vi "4Pi Focus Lock - Setup Camera.vi"(0 "Camera Notifier Name":string) -> (8 "Canceled?":bool)   [LabVIEW 2016]
uses:
  <vilib>/Utility/miscctls.llb/LVPointTypeDef.ctl
  Device Library/Cameras/Camera Controls/Generic Camera ROI.ctl
  Device Library/Cameras/Camera Controls/Generic Camera Actions.ctl
  4Pi Focus Lock Controls/4Pi Focus Lock - Camera Settings.ctl
panel:
  out "ROI Size":string
  in  "Exposure Time (ms)":dbl
  in  "Tool Selection":enum32{"Zoom Tool", "ROI Tool", "Pan Tool"}(radio)
  in  "Cancel":bool
  in  "Done":bool
  out "Camera Display":T1(plugin-control)
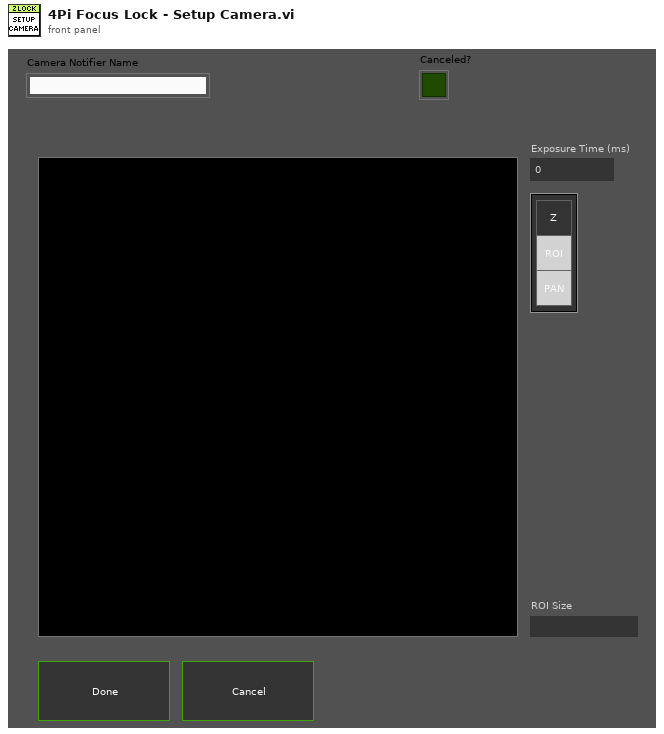
[diagram p1: front panel]
types:
  T1 = typedef "IMAQ Image.ctl" = refnum<image>
  T2 = typedef "Generic Camera Actions.ctl" = enum16{"Status", "Live Preview", "Capture", "Abort", "Set Exposure Time (s)", "Get Exposure Time (s)", "Record Settings", "Set ROI", "Get ROI", "Defect Correction On/Off", "Cooler On/Off", "Fan On/Off", "Quit"}
  T3 = typedef "Generic Camera ROI.ctl" = cluster{"H_Offset":u16, "V_Offset":u16, "H_Width":u16, "V_Width":u16}
  T4 = enum16{"Always On", "Always Off", "Off While Running"}
  T5 = typedef "LVPointTypeDef.ctl" = cluster{"Horizontal":i16, "Vertical":i16}
  T6 = typedef "LVRectTypeDef.ctl" = cluster{"Left":i16, "Top":i16, "Right":i16, "Bottom":i16}
  T7 = typedef "LVBoundsTypeDef.ctl" = cluster{"Width":u32, "Height":u32}
  T8 = typedef "4Pi Focus Lock - Camera Settings.ctl" = cluster{"Exposure Time (s)":dbl, "H Offset":u16, "V Offset":u16, "H Width":u16, "V Width":u16}
  T9 = cluster{"Global Rectangle":i32[], "Contours":cluster{"Contour Type":u32, "ROI Type":u32, "Points":i32[]}[]}
  T10 = cluster{"Contour Type":u32, "ROI Type":u32, "Points":i32[]}[]
  T11 = cluster{"Contour Type":u32, "ROI Type":u32, "Points":i32[]}
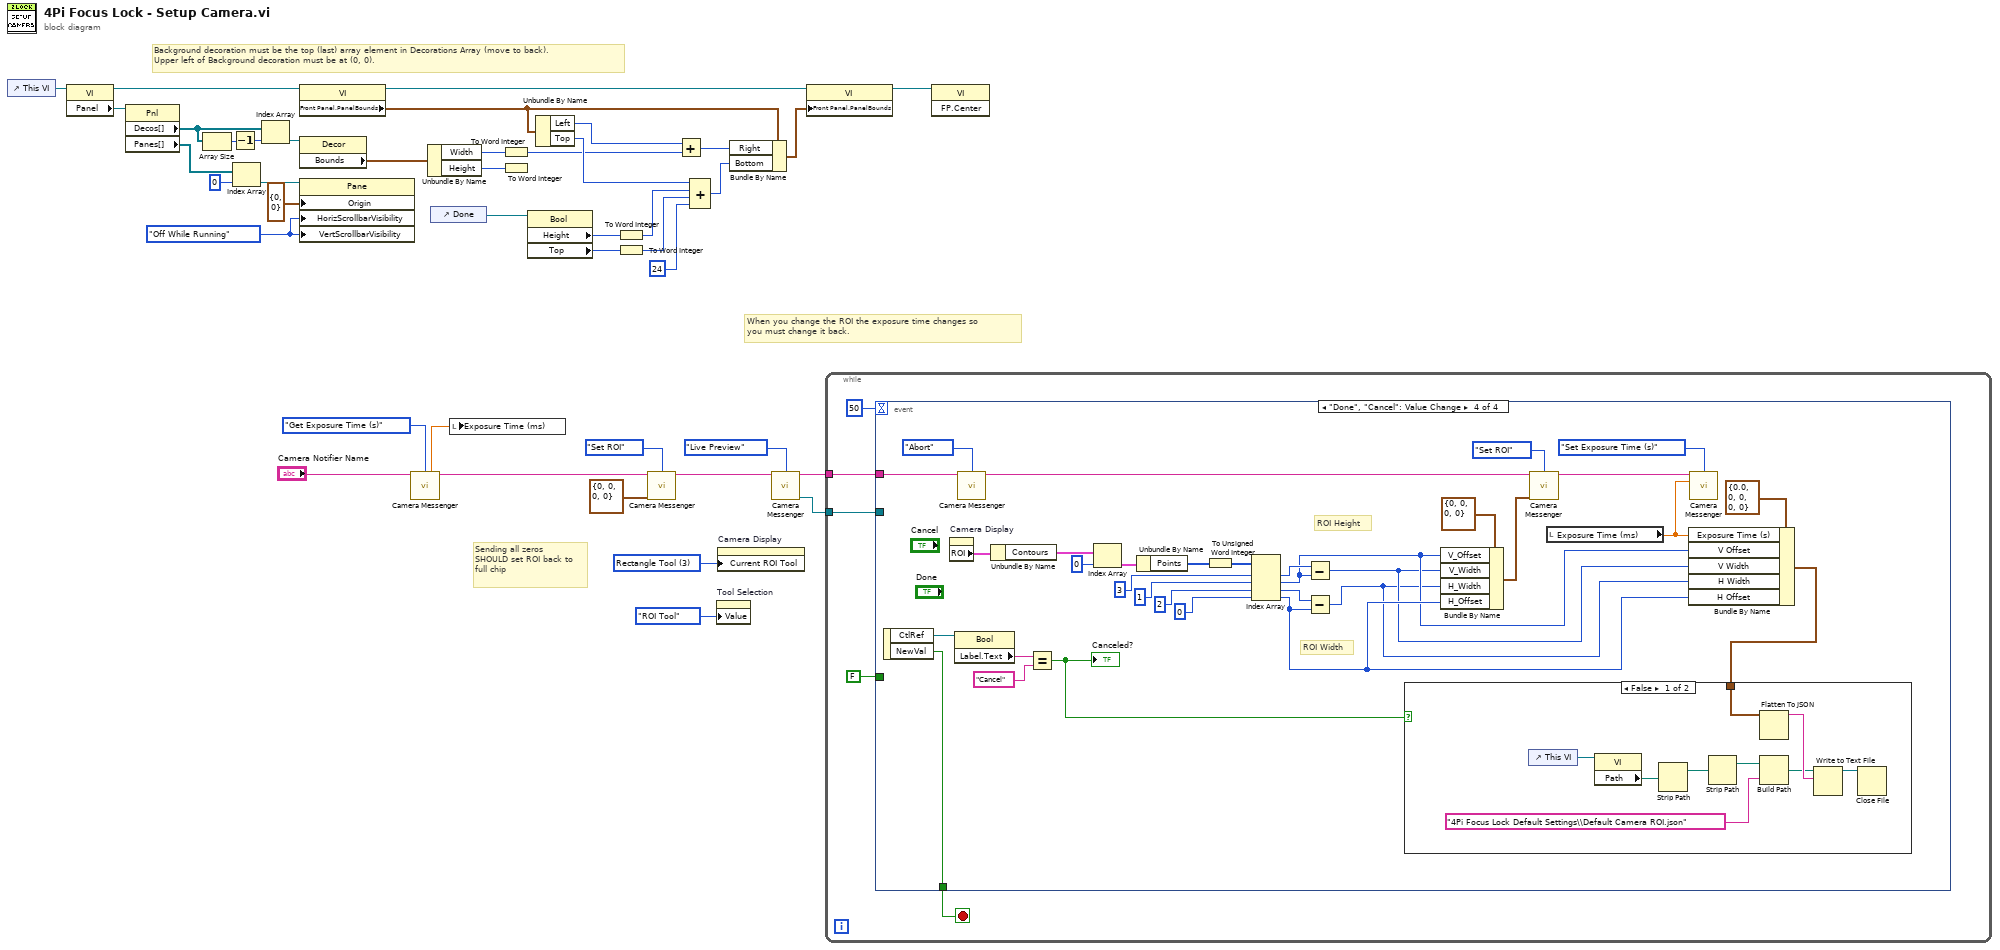
[diagram p0: block diagram]
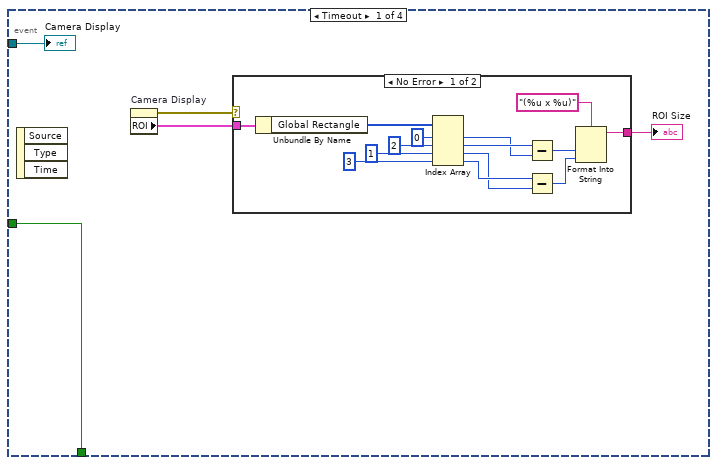
[diagram p2: hidden frame]
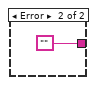
[diagram p3: hidden frame]
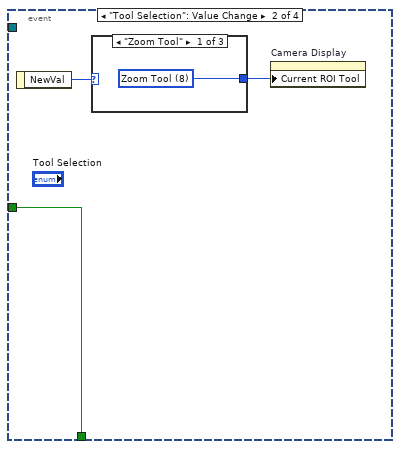
[diagram p4: hidden frame]
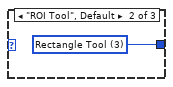
[diagram p5: hidden frame]
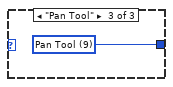
[diagram p6: hidden frame]
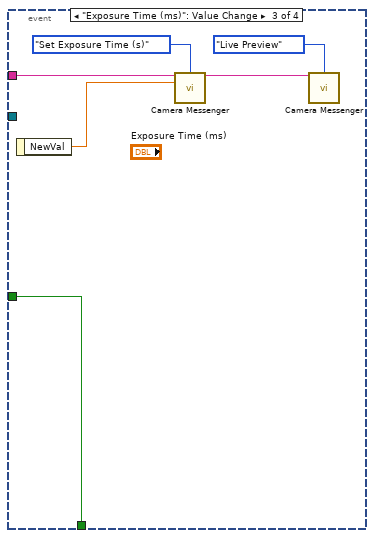
[diagram p7: hidden frame]
diagram:
  w23 = T4."Off While Running" ("Vertical Scrollbar Visibility")
  w42 = u32 3 items=["Zoom Tool"=8, "Selection Tool"=0, "Pan Tool"=9, "Point Tool"=1, "Line Tool"=2, "Rectangle Tool"=3, "Rotated Rectangle Tool"=12, "Polyline Tool"=10, "Polygon Tool"=5, "Freehand Tool"=11, "Closed Freehand Tool"=6, "Ellipse Tool"=4, "Annulus Tool"=7] ("Current ROI Tool")
  # "Background decoration must be the top (last) array element in Decorations Array (move to back).\nUpper left of Background decoration must be at (0, 0)."
  # "When you change the ROI the exposure time changes so\nyou must change it back."
  # "Sending all zeros SHOULD set ROI back to full chip"
  n1 = control-ref of="This VI"() -> (w15:refnum<vi>)
  n2 = property class="VI"(reference=w15) -> (reference out=w24:refnum<vi>, "Panel"=w16:refnum<vi>)  [unwired: 1 in, 1 out]
  n3 = property class="Pnl"(reference=w16) -> ("Decos[]"=w14:refnum<vi>[], "Panes[]"=w20:refnum<vi>[])  [unwired: 1 in, 2 out]
  n4 = Array Size(array=w14) -> (size(s)=w12:i32)
  n5 = Decrement(x=w12) -> (x-1=w13:i32)
  n6 = Index Array(array=w20, index=0) -> (element=w19:refnum<vi>)
  n7 = Index Array(array=w14, index=w13) -> (element=w22:refnum<vi>)
  n8 = property class="VI"(reference=w24) -> (reference out=w26:refnum<vi>, "Front Panel.PanelBounds"=w27:T6)  [unwired: 1 in, 1 out]
  n9 = property class="Decor"(reference=w22) -> ("Bounds"=w25:T7)  [unwired: 1 in, 2 out]
  n10 = property class="Pane"(reference=w19, "Origin"=T5 {"Horizontal"=0, "Vertical"=0}, "HorizScrollbarVisibility"=w23, "VertScrollbarVisibility"=w23) -> ()  [unwired: 1 in, 2 out]
  n11 = call "Camera Messenger.vi"("Notifier Name"="Camera Notifier Name", "General Camera Actions"=Generic_Camera_Actions."Get Exposure Time (s)") -> ("Current Exposure Time (s)"=w8:dbl, "Notifier Name Dup"=w7:string)  [unwired: 8 in, 4 out]
  n12 = Unbundle By Name(w25) -> ("Width"=w30:u32, "Height"=w33:u32)
  n13 = control-ref of="Done"() -> (w17:refnum<vi>)
  n14 = local write "Exposure Time (ms)"(w8) -> ()
  n15 = To Word Integer(number=w30) -> (16bit integer=w32:i16)
  n16 = To Word Integer(number=w33) -> ()  [unwired: 1 out]
  n17 = property class="Bool"(reference=w17) -> ("Height"=w35:u32, "Top"=w36:i32)  [unwired: 1 in, 2 out]
  n18 = Unbundle By Name(w27) -> ("Left"=w29:i16, "Top"=w40:i16)
  n19 = To Word Integer(number=w35) -> (16bit integer=w38:i16)
  n20 = To Word Integer(number=w36) -> (16bit integer=w39:i16)
  n21 = call "Camera Messenger.vi"("Notifier Name"=w7, "General Camera Actions"=Generic_Camera_Actions."Set ROI", "Camera ROI"=T3 {"H_Offset"=0, "V_Offset"=0, "H_Width"=0, "V_Width"=0} ("General Camera ROI")) -> ("Notifier Name Dup"=w4:string)  [unwired: 7 in, 5 out]
  n22 = Add(x=w29, y=w32) -> (x+y=w31:i16)
  n23 = Compound Arithmetic op=ADD(w40, w38, w39, i16 24 ("y")) -> (w34:i16)
  n24 = property on="Tool Selection" class="RadioBtnsControl (strict)"("Value"=enum32{"Zoom Tool", "ROI Tool", "Pan Tool"}."ROI Tool" ("Tool Selection")) -> ()  [unwired: 2 in, 2 out]
  n25 = property on="Camera Display" class="ImageControl"("Current ROI Tool"=w42) -> ()  [unwired: 2 in, 2 out]
  n26 = Bundle By Name(cluster=w27, "Right"=w31, "Bottom"=w34) -> (w28:T6)
  n27 = call "Camera Messenger.vi"("Notifier Name"=w4, "General Camera Actions"=Generic_Camera_Actions."Live Preview") -> ("Notifier Name Dup"=w3:string, "Image Ref"=w1:T1)  [unwired: 8 in, 4 out]
  n28 = property class="VI"(reference=w26, "Front Panel.PanelBounds"=w28) -> (reference out=w11:refnum<vi>)  [unwired: 1 in, 1 out]
  n29 = while {
    tunnel: w1 -> [w45]
    tunnel: w3 -> [w43]
    stop <- w47 stop-if-true
    n30 = event shown="[3] \"Done\", \"Cancel\": Value Change" {
      selector: _ -> [_ _ _ _]
      dyn-events: _ -> [_ _ _ _]
      timeout: 50 -> [_ _ _ _]
      tunnel: [w52 w70 w79 w108] -> w47
      tunnel: FALSE -> [w52 w70 w79 _]
      tunnel: w45 -> [w51 _ _ _]
      tunnel: w43 -> [_ _ w78 w96]
      event Timeout {
        n31 = event-data() -> ()  [unwired: 1 in, 3 out]
        n32 = property on="Camera Display" class="ImageControl"() -> (error out=w49:errorcluster, "ROI"=w50:T9)  [unwired: 2 in, 1 out]
        n33 = case shown="No Error" w49 {
          tunnel: w50 -> [w57 _]
          tunnel: [w53 ""] -> w48
          frame No Error {
            n34 = Unbundle By Name(w57) -> ("Global Rectangle"=w66:i32[])
            n35 = Index Array(array=w66, index #1=0 ("index"), index #2=2 ("index"), index #3=1 ("index"), index #4=3 ("index")) -> (element #1=w60:i32, element #2=w61:i32, element #3=w58:i32, element #4=w59:i32)
            n36 = Subtract(x=w61, y=w60) -> (x-y=w55:i32)
            n37 = Subtract(x=w59, y=w58) -> (x-y=w54:i32)
            n38 = Format Into String(format string="(%u x %u)", w55, w54) -> (resulting string=w53:string)  [unwired: 2 in, 1 out]
          }
          frame Error {
          }
        }
        "ROI Size" <- w48
        "Camera Display" <- w51
      }
      event "Tool Selection": Value Change {
        n39 = event-data() -> ("NewVal"=w69:enum32{"Zoom Tool", "ROI Tool", "Pan Tool"})  [unwired: 1 in]
        n40 = case shown="\"Zoom Tool\"" w69 {
          tunnel: [w71 w72 w73] -> w68
          frame "Zoom Tool" {
            w71 = u32 8 items=["Zoom Tool"=8, "Selection Tool"=0, "Pan Tool"=9, "Point Tool"=1, "Line Tool"=2, "Rectangle Tool"=3, "Rotated Rectangle Tool"=12, "Polyline Tool"=10, "Polygon Tool"=5, "Freehand Tool"=11, "Closed Freehand Tool"=6, "Ellipse Tool"=4, "Annulus Tool"=7] ("Current ROI Tool")
          }
          frame "ROI Tool", Default {
            w72 = u32 3 items=["Zoom Tool"=8, "Selection Tool"=0, "Pan Tool"=9, "Point Tool"=1, "Line Tool"=2, "Rectangle Tool"=3, "Rotated Rectangle Tool"=12, "Polyline Tool"=10, "Polygon Tool"=5, "Freehand Tool"=11, "Closed Freehand Tool"=6, "Ellipse Tool"=4, "Annulus Tool"=7] ("Current ROI Tool")
          }
          frame "Pan Tool" {
            w73 = u32 9 items=["Zoom Tool"=8, "Selection Tool"=0, "Pan Tool"=9, "Point Tool"=1, "Line Tool"=2, "Rectangle Tool"=3, "Rotated Rectangle Tool"=12, "Polyline Tool"=10, "Polygon Tool"=5, "Freehand Tool"=11, "Closed Freehand Tool"=6, "Ellipse Tool"=4, "Annulus Tool"=7] ("Current ROI Tool")
          }
        }
        n41 = property on="Camera Display" class="ImageControl"("Current ROI Tool"=w68) -> ()  [unwired: 2 in, 2 out]
      }
      event "Exposure Time (ms)": Value Change {
        n42 = event-data() -> ("NewVal"=w76:dbl)  [unwired: 1 in]
        n43 = call "Camera Messenger.vi"("Notifier Name"=w78, "General Camera Actions"=Generic_Camera_Actions."Set Exposure Time (s)", "Exposure Time (s)"=w76) -> ("Notifier Name Dup"=w75:string)  [unwired: 7 in, 5 out]
        n44 = call "Camera Messenger.vi"("Notifier Name"=w75, "General Camera Actions"=Generic_Camera_Actions."Live Preview") -> ()  [unwired: 8 in, 6 out]
      }
      event "Done", "Cancel": Value Change {
        # "ROI Width"
        # "ROI Height"
        n45 = event-data() -> ("CtlRef"=w111:refnum<vi>, "NewVal"=w108:bool)  [unwired: 1 in]
        n46 = property on="Camera Display" class="ImageControl"() -> ("ROI"=w104:T9)  [unwired: 2 in, 2 out]
        n47 = property class="Bool"(reference=w111) -> ("Label.Text"=w110:string)  [unwired: 1 in, 2 out]
        n48 = call "Camera Messenger.vi"("Notifier Name"=w96, "General Camera Actions"=Generic_Camera_Actions."Abort") -> ("Notifier Name Dup"=w93:string)  [unwired: 8 in, 5 out]
        n49 = Unbundle By Name(w104) -> ("Contours"=w103:T10)
        n50 = Equal?(x=w110, y="Cancel") -> (x = y?=w80:bool)
        "Canceled?" <- w80
        n51 = Index Array(array=w103, index=0) -> (element=w102:T11)
        n52 = Unbundle By Name(w102) -> ("Points"=w105:i32[])
        n53 = To Unsigned Word Integer(number=w105) -> (unsigned 16bit integer=w86:u16[])
        n54 = Index Array(array=w86, index #1=3 ("index"), index #2=1 ("index"), index #3=2 ("index"), index #4=0 ("index")) -> (element #1=w107:u16, element #2=w84:u16, element #3=w106:u16, element #4=w85:u16)
        n55 = Subtract(x=w107, y=w84) -> (x-y=w83:u16)
        n56 = Subtract(x=w106, y=w85) -> (x-y=w82:u16)
        n57 = Bundle By Name(cluster=T3 {"H_Offset"=0, "V_Offset"=0, "H_Width"=0, "V_Width"=0} ("General Camera ROI"), "V_Offset"=w84, "V_Width"=w83, "H_Width"=w82, "H_Offset"=w85) -> (w92:T3)
        n58 = call "Camera Messenger.vi"("Notifier Name"=w93, "General Camera Actions"=Generic_Camera_Actions."Set ROI", "Camera ROI"=w92) -> ("Notifier Name Dup"=w90:string)  [unwired: 7 in, 5 out]
        n59 = local read "Exposure Time (ms)"() -> (w87:dbl)
        n60 = Bundle By Name(cluster=T8 {"Exposure Time (s)"=0.0, "H Offset"=0, "V Offset"=0, "H Width"=0, "V Width"=0} ("Camera Settings"), "Exposure Time (s)"=w87, "V Offset"=w84, "V Width"=w83, "H Width"=w82, "H Offset"=w85) -> (w81:T8)
        n61 = case shown="False" w80 {
          tunnel: w81 -> [w112 _]
          frame False {
            n62 = control-ref of="This VI"() -> (w115:refnum<vi>)
            n63 = property class="VI"(reference=w115) -> ("Path"=w114:path)  [unwired: 1 in, 2 out]
            n64 = Strip Path(path=w114) -> (stripped path=w116:path)  [unwired: 1 out]
            n65 = Strip Path(path=w116) -> (stripped path=w117:path)  [unwired: 1 out]
            n66 = Flatten To JSON(anything=w112) -> (JSON string=w119:string)  [unwired: 2 in, 1 out]
            n67 = Build Path(base path=w117, name or relative path="4Pi Focus Lock Default Settings\\Default Camera ROI.json") -> (appended path=w113:path)
            n68 = Write to Text File(file (use dialog)=w113, text=w119) -> (refnum out=w120:refnum<file>)  [unwired: 2 in, 2 out]
            n69 = Close File(refnum=w120) -> ()  [unwired: 1 in, 2 out]
          }
          frame True {
          }
        }
        n70 = call "Camera Messenger.vi"("Notifier Name"=w90, "General Camera Actions"=Generic_Camera_Actions."Set Exposure Time (s)", "Exposure Time (s)"=w87) -> ()  [unwired: 7 in, 6 out]
      }
    }
  }
  n71 = invoke class="VI" method="FP.Center"(reference=w11) -> ()  [unwired: 2 in, 3 out]
